vi "Set volume.vi"(7 "[x]":T1, 8 "error in (no error)":errorcluster, 10 "Volume (array)":dbl[](array[numeric]), 11 "Serial Port in":refnum<visa-resource-name>) -> (0 "error out":errorcluster, 3 "Serial Port out":refnum<visa-resource-name>)   [LabVIEW 2016, in "Chemyx_Syringe_Pump_driver.lvlib"]
doc: "Sets the volumes of the syringe oeprations.\n\nVolume is an array of double float. Units are those defined by the set units operation.\n\nInfusions are accomplished using positive and withdraws are accomplished using negative volumes."
uses:
  Chemyx_Syringe_Pump_driver.lvlib
  _private/Control/Control Mode.ctl
panel:
  # "Sets the diameter of the syringe"
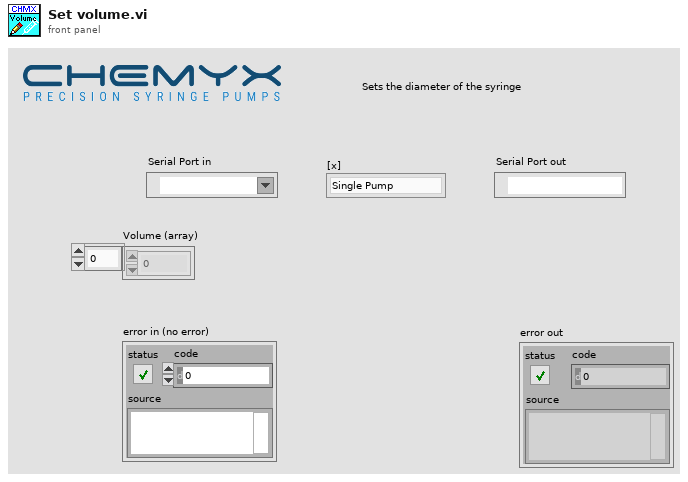
[diagram p1: front panel]
types:
  T1 = typedef "Chemyx_Syringe_Pump_driver.lvlib/Control Mode.ctl" = enum16{"Single Pump", "Pump Chanel 1", "Pump Channel 2", "Cycle Mode"}
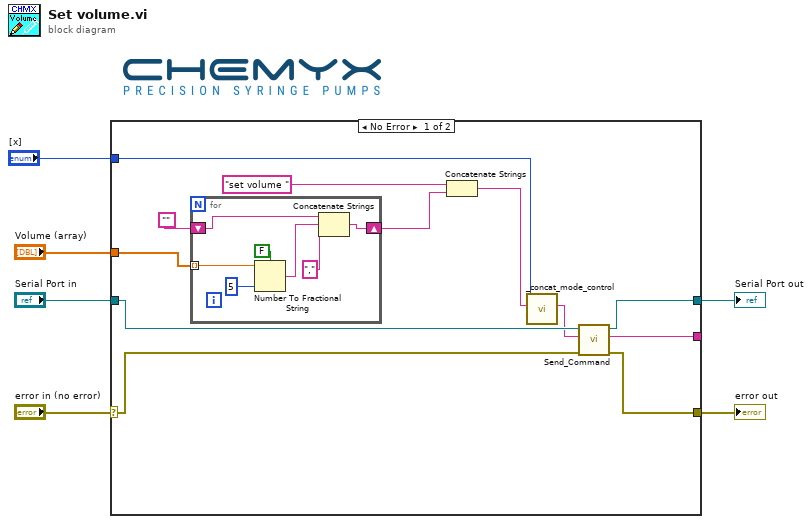
[diagram p0: block diagram]
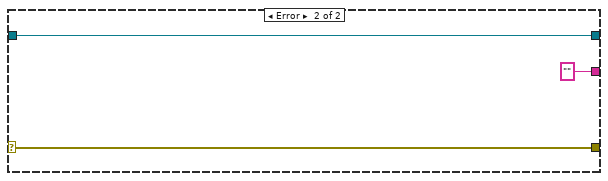
[diagram p2: hidden frame]
diagram:
  n1 = case shown="No Error" "error in (no error)" {
    selector: "error in (no error)" -> [w17 w28]
    tunnel: "Serial Port in" -> [w18 w27]
    tunnel: [w16 w28] -> w4
    tunnel: [w15 w27] -> w3
    tunnel: "Volume (array)" -> [w13 _]
    tunnel: [w12 "" ("Read buffer")] -> _
    tunnel: "[x]" -> [w7 _]
    frame No Error {
      n2 = for {
        tunnel: w13 -> [w25] mode=indexing
        shift-right: [w22] -> w10
        shift-left: "" -> [w21]
        n3 = Number To Fractional String(use system decimal point (T)=FALSE, number=w25, precision (6)=i16 5) -> (F-format string=w20:string)  [unwired: 1 in]
        n4 = Concatenate Strings(w21, w20, "," ("string")) -> (w22:string)
      }
      n5 = Concatenate Strings("set volume ", w10) -> (w9:string)
      n6 = call "_concat_mode_control.vi"("write buffer"=w9, "[x]"=w7) -> ("write buffer out"=w8:string)  [unwired: 9 in]
      n7 = call "Send_Command.vi"("error in (no error)"=w17, "write buffer"=w8, "Serial Port in"=w18) -> ("error out"=w16:errorcluster, "Read buffer"=w12:string, "VISA Refnum out"=w15:refnum<visa-resource-name>)  [unwired: 6 in]
    }
    frame Error {
    }
  }
  "error out" <- w4
  "Serial Port out" <- w3
